vi "Upload VASP File2.vi"(8 "Upload DOS?":bool, 10 "connection reference":T1, 11 "Directory to upload":path=path "C:/Users/Chris B/Documents/Ab Initio/Vasp Calculations/Batch4_20130519/1_Again") -> (3 "IDs":T2)   [LabVIEW 2010]
uses:
  <vilib>/addons/database/NI_Database_API.lvlib
  <vilib>/Analysis/NI_AALBase.lvlib
  <vilib>/Analysis/NI_AALPro.lvlib
  <vilib>/Analysis/_algsub.llb/Real Vector Norm.vi
  <vilib>/Utility/error.llb/DialogType.ctl
  <vilib>/addons/database/Connection.llb/DB Tools Open Connec (Path).vi
  <vilib>/addons/database/Connection.llb/Conn Get Properties.vi
  <vilib>/Utility/file.llb/Read From Spreadsheet File (string).vi
  <vilib>/Analysis/baseanly.llb/Real Dot Product.vi
  <vilib>/addons/database/Connection.llb/Conn ObjectReference.ctl
panel:
  out "INCAR ID":string
  in  "Show Errors?":bool
  out "README":bool
  out "# of atoms":i32
  out "CONTCAR":T3
  out "POSCAR":T3
  out "OUTCAR":bool
  out "DOSCAR":bool
  out "CONTCAR":bool
  out "POSCAR":bool
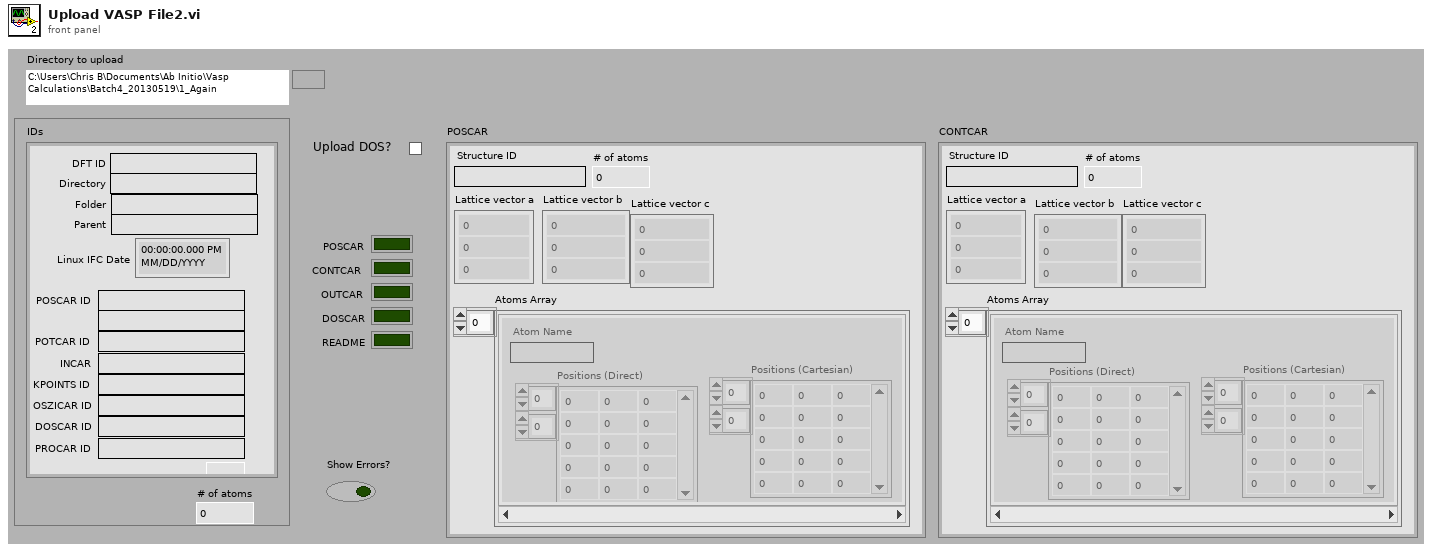
[diagram p1: front panel]
types:
  T1 = typedef "NI_Database_API.lvlib/Conn ObjectReference.ctl" = refnum<k1>
  T2 = cluster{"DFT ID":string, "Directory":string, "Folder":string, "Parent":string, "Linux IFC Date":timestamp, "POSCAR ID":string, "CONTCAR ID":string, "POTCAR ID":string, "INCAR":string, "KPOINTS ID":string, "OSZICAR ID":string, "DOSCAR ID":string, "PROCAR ID":string, "Calc time (Hrs)":dbl}
  T3 = cluster{"Structure ID":string, "Lattice vector a":dbl[], "Lattice vector b":dbl[], "Lattice vector c":dbl[], "Atoms Array":cluster{"Atom Name":string, "Positions (Direct)":dbl[][], "Positions (Cartesian)":dbl[][]}[], "# of atoms":i32}
  T4 = cluster{"Command":string, "Value":string, "Comment":string}[]
  T5 = cluster{"INCAR ID":string, "IBRION":string, "ISIF":string, "ISMEAR":string, "ISPIN":string, "Net Charge":i32}
  T6 = cluster{"INCAR ID":string, "Command":string, "Value":string, "Comment":string}
  T7 = typedef "DialogType.ctl" = u16
  T8 = cluster{"Structure Name":string, "Lattice vector a":dbl[], "Lattice vector b":dbl[], "Lattice vector c":dbl[], "Atoms Array":cluster{"Atom Name":string, "Positions (Direct)":dbl[][], "Positions (Cartesian)":dbl[][]}[], "# of atoms":i32}
  T9 = cluster{"MD5 message-digest":string, string, "name":string, "name":string, "Relaxation Time":timestamp, "Structure ID":string, "Structure ID":string, "MD5 message-digest":string, "INCAR ID":string, "MD5 message-digest":string, "MD5 message-digest":string, "MD5 message-digest":string, "MD5 message-digest":string, "Calc Time (Hrs)":dbl}
  T10 = cluster{"Atom Name":string, "Positions (Direct)":dbl[][], "Positions (Cartesian)":dbl[][]}[]
  T11 = cluster{"[0]":string, "[1]":string, "[2]":string, "[3]":string, "[4]":string, "[5]":string, "[6]":string, "[7]":string, "[8]":string, "[9]":string, "[10]":string, "[11]":string, "[12]":string, "[13]":string, "[14]":string, "[15]":string, "[16]":string, "[17]":string}
  T12 = cluster{"Structure ID":string, "Atom Name":string, "Numeric":dbl, "Numeric":dbl, "Numeric":dbl}
  T13 = cluster{"POTCAR ID":string, "trimmed string":string}
  T14 = cluster{"OSZICAR data":cluster{"Total Free Energy (eV)":dbl, "E0 at Sigma=0 (eV)":dbl, "dE (eV)":dbl, "Electronic Relaxation":dbl[][]}[], "Ionic Relaxation Energies Array (eV)":dbl[], "Bulk Formation Energies Array (eV)":dbl[]}
  T15 = cluster{"Final Energy (eV)":dbl, "Final Energy/atom (eV/atom)":dbl, "Total Formation Energy (eV)":dbl}
  T16 = cluster{"OSZICAR ID":string, "Final Energy (eV)":dbl, "Final Energy/atom (eV/atom)":dbl, "Total Formation Energy (eV)":dbl, i32}
  T17 = cluster{"Energy (eV)":dbl[], "Total DOS":dbl[], "Integrated DOS":dbl[]}
  T18 = cluster{"Fermi Level (eV)":dbl, "# States":dbl, "Density of Valence Band":dbl, "Density of Condution Band":dbl}
  T19 = cluster{"DOSCAR ID":string, "Energy (eV)":dbl[], "Total DOS":dbl[], "Integrated DOS":dbl[], void}
  T20 = cluster{"DOSCAR ID":string, i32, void, void, void}
  T21 = cluster{"DFT ID":string, "String":string, "String":string}
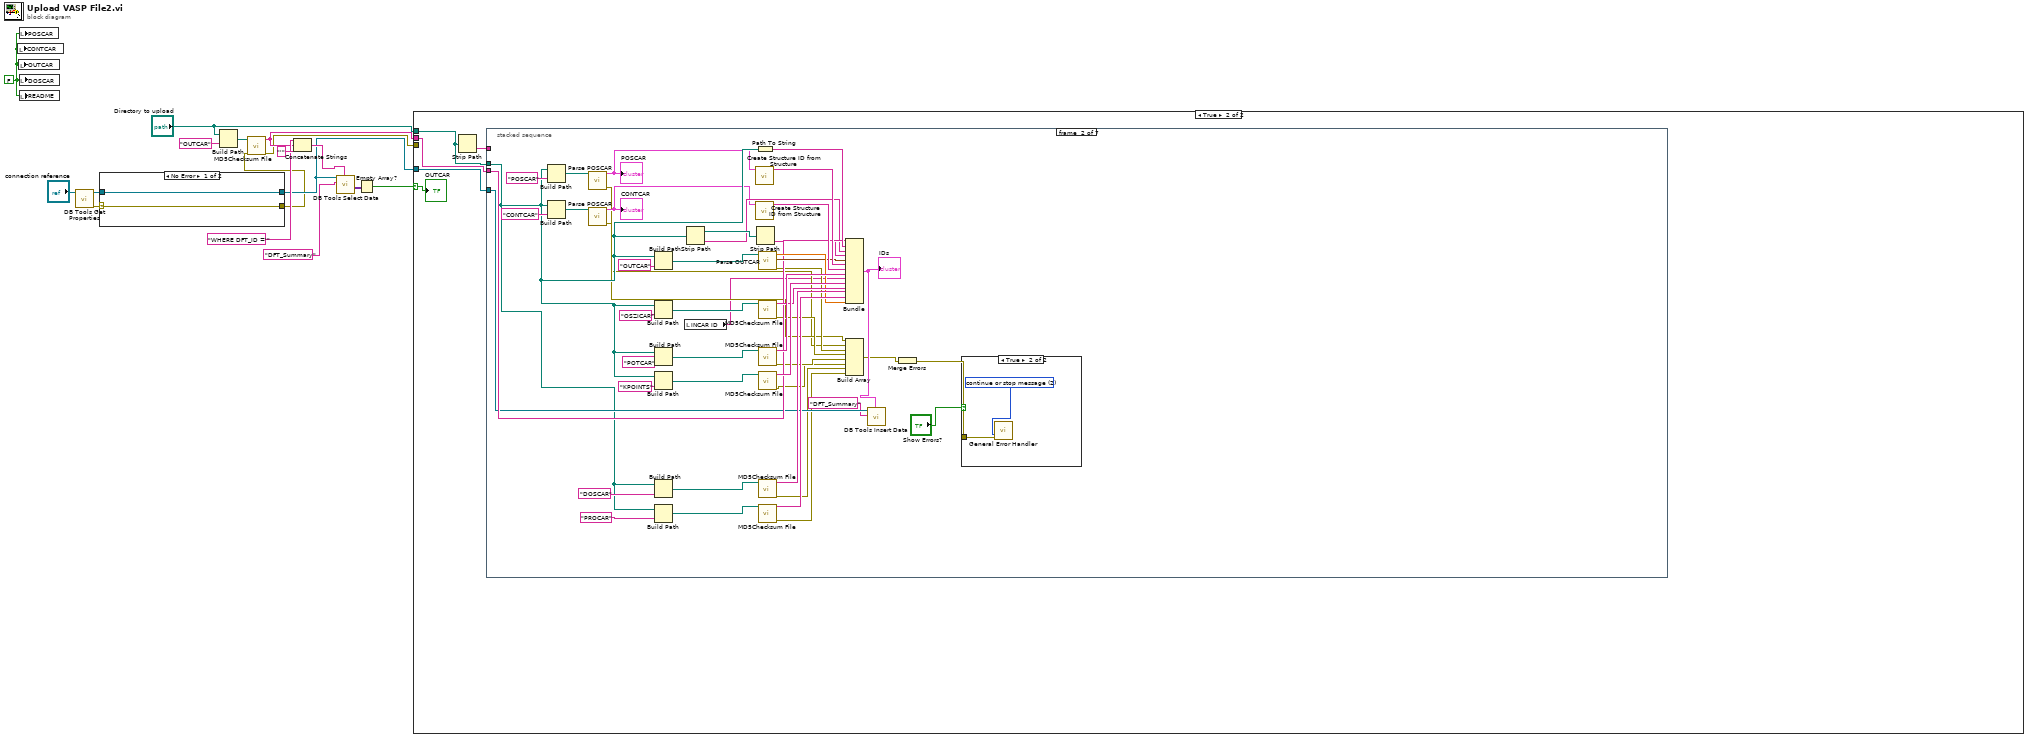
[diagram p0: block diagram]
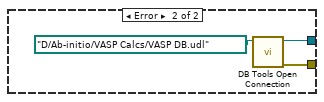
[diagram p2: hidden frame]
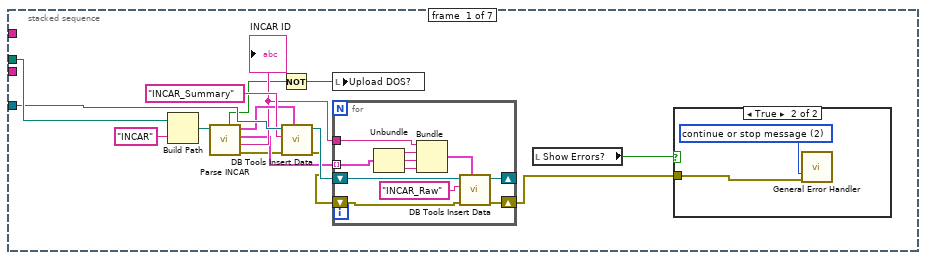
[diagram p4: hidden frame]
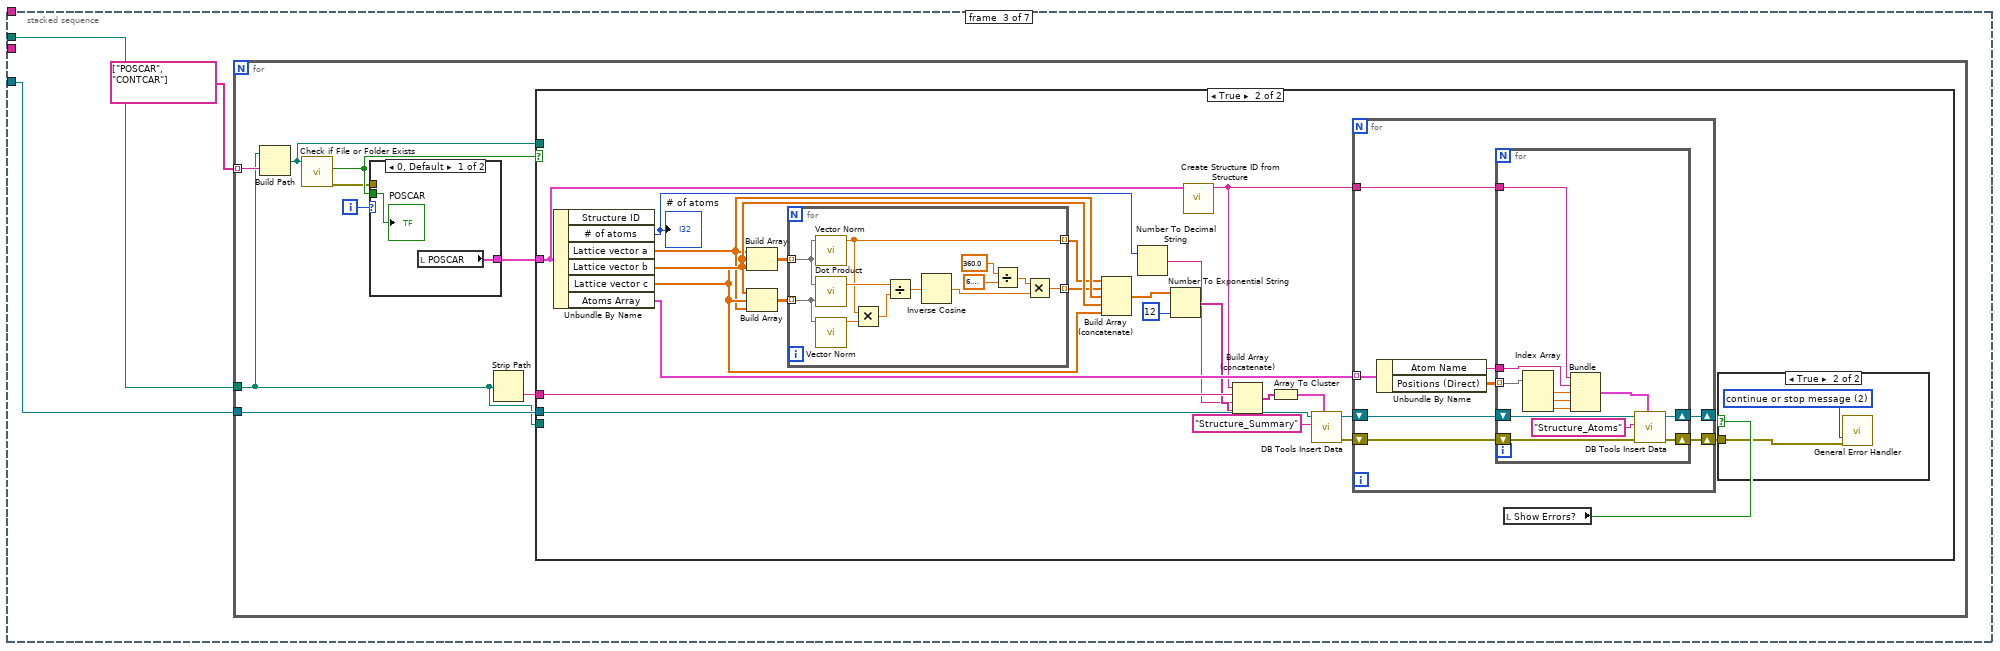
[diagram p7: hidden frame]
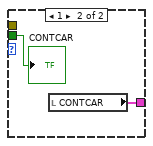
[diagram p10: hidden frame]
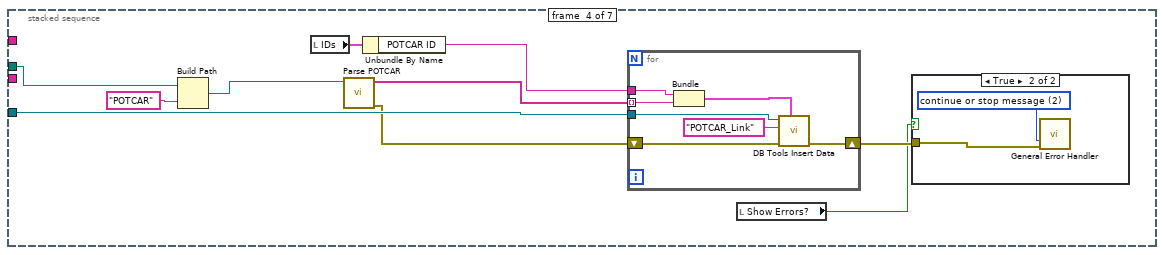
[diagram p11: hidden frame]
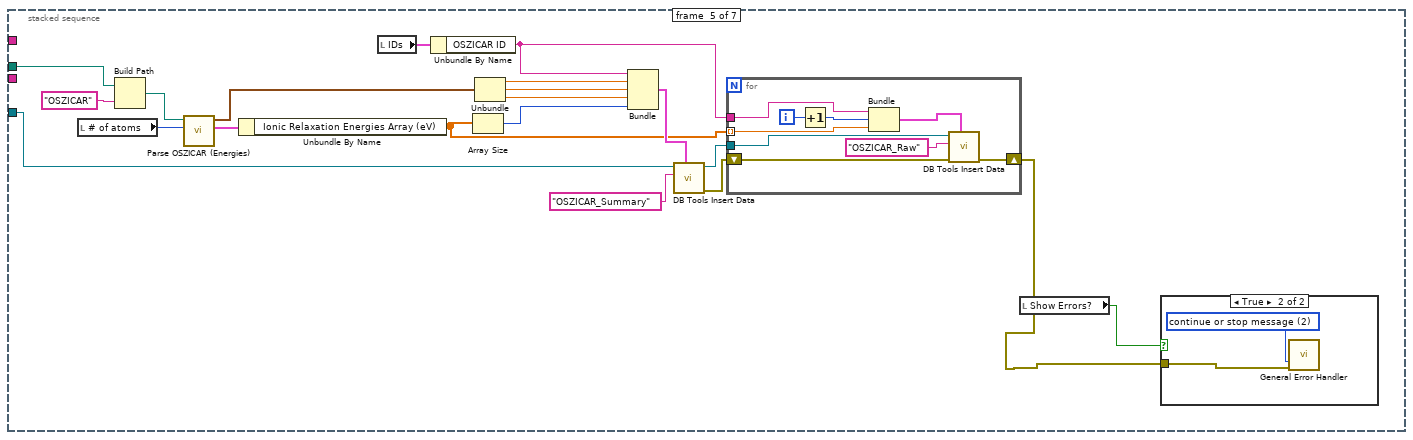
[diagram p13: hidden frame]
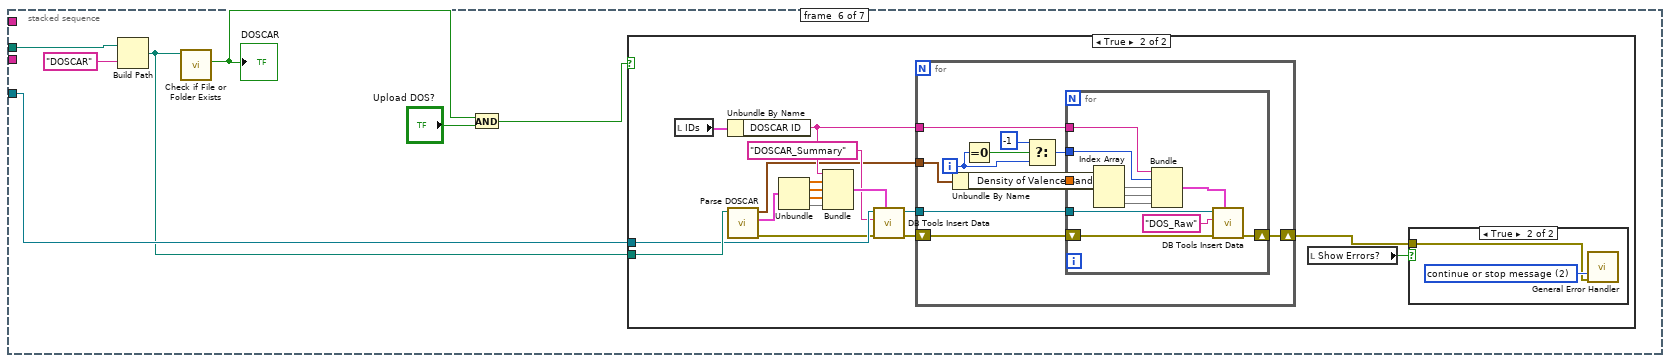
[diagram p15: hidden frame]
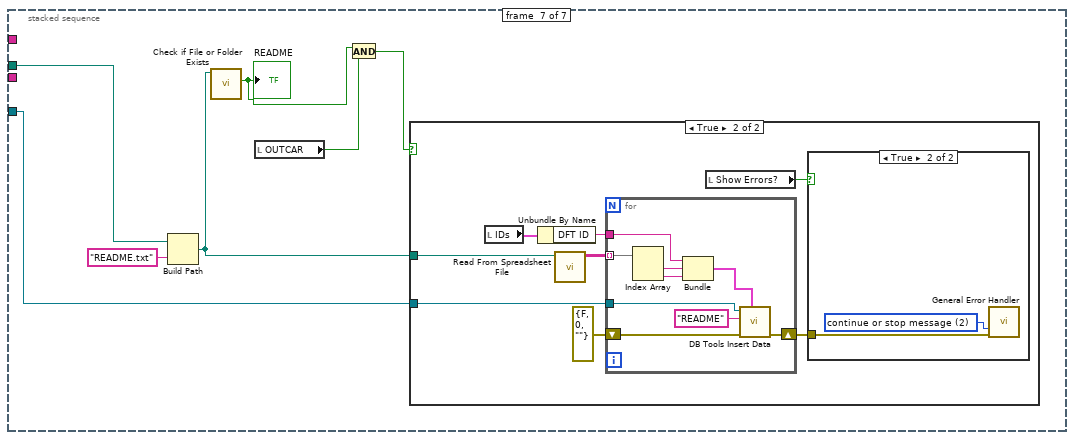
[diagram p18: hidden frame]
diagram:
  w8 = FALSE
  n1 = local write "CONTCAR"(w8) -> ()
  n2 = local write "OUTCAR"(w8) -> ()
  n3 = local write "POSCAR"(w8) -> ()
  n4 = local write "DOSCAR"(w8) -> ()
  n5 = local write "README"(w8) -> ()
  n6 = call-poly <vilib>:"DB Tools Get Properties.vi"("connection reference"="connection reference") -> ("error out"=w5:errorcluster, "connection reference out"=w4:T1)  [unwired: 4 in, 1 out]
  n7 = case shown="No Error" w5 {
    selector: w5 -> [w18 _]
    tunnel: w4 -> [w19 _]
    tunnel: [w19 w22] -> w3
    tunnel: [w18 w20] -> w2
    frame No Error {
    }
    frame Error {
      n8 = call-poly <vilib>:"DB Tools Open Connection.vi"("connection information"=path "D:/Ab-initio/VASP Calcs/VASP DB.udl" ("UDL")) -> ("error out"=w20:errorcluster, "connection reference"=w22:T1)  [unwired: 7 in]
    }
  }
  n9 = Build Path(base path="Directory to upload", name or relative path="OUTCAR") -> (appended path=w13:path)
  n10 = call <vilib>:"MD5Checksum File.vi"("error in (no error)"=w2, "Path"=w13) -> ("error out"=w7:errorcluster, "MD5 message-digest"=w11:string)  [unwired: 8 in]
  n11 = Concatenate Strings("WHERE DFT_ID ='" ("string"), w11, "'" ("string")) -> (w17:string)
  n12 = call <vilib>:"DB Tools Select Data.vi"("condition"=w17, "table"="DFT_Summary", "connection reference"=w3) -> ("data"=w1:variant[][])  [unwired: 3 in, 2 out]
  n13 = Empty Array?(array=w1) -> (empty?=w9:bool)
  n14 = case shown="True" w9 {
    selector: w9 -> [_ w23]
    tunnel: w11 -> [_ w26]
    tunnel: w3 -> [_ w25]
    tunnel: "Directory to upload" -> [_ w24]
    tunnel: w7 -> [_ _]
    frame False {
    }
    frame True {
      n15 = Strip Path(path=w24) -> (name=w27:string)  [unwired: 1 out]
      n16 = stacked-sequence {
        tunnel: w24 -> [w42 w75 w108 w189 w217 w236 w282]
        tunnel: w25 -> [w38 w76 w107 w183 w206 w235 w281]
        tunnel: w27 -> [_ _ _ _ _ _ _]
        tunnel: w26 -> [_ w77 _ _ _ _ _]
        frame #0 {
          n17 = Build Path(base path=w42, name or relative path="INCAR") -> (appended path=w40:path)
          n18 = call "Parse INCAR.vi"("INCAR File"=w40) -> ("error out"=w31:errorcluster, "INCAR ID"=w34:string, "INCAR Raw Commands"=w33:T4, "INCAR Summary"=w35:T5, "Allow Relaxation?"=w32:bool)  [unwired: 6 in]
          "INCAR ID" <- w34
          n19 = Not(x=w32) -> (.not. x?=w39:bool)
          n20 = call <vilib>:"DB Tools Insert Data.vi"("data"=w35, "error in (no error)"=w31, "table"="INCAR_Summary", "connection reference"=w38) -> ("error out"=w29:errorcluster, "connection reference out"=w37:T1)  [unwired: 6 in]
          n21 = local write "Upload DOS?"(w39) -> ()
          n22 = for {
            tunnel: w33 -> [w55] mode=indexing
            tunnel: w34 -> [w48]
            shift-right: [w53] -> _
            shift-left: w37 -> [w54]
            shift-right: [w46] -> w28
            shift-left: w29 -> [w45]
            n23 = Unbundle(w55) -> ("Command"=w52:string, "Value"=w51:string, "Comment"=w50:string)
            n24 = Bundle("INCAR ID"=w48, "Command"=w52, "Value"=w51, "Comment"=w50) -> (w49:T6)  [unwired: 1 in]
            n25 = call <vilib>:"DB Tools Insert Data.vi"("data"=w49, "error in (no error)"=w45, "table"="INCAR_Raw", "connection reference"=w54) -> ("error out"=w46:errorcluster, "connection reference out"=w53:T1)  [unwired: 6 in]
          }
          n26 = local read "Show Errors?"() -> (w30:bool)
          n27 = case shown="True" w30 {
            tunnel: w28 -> [_ w44]
            frame False {
            }
            frame True {
              w43 = T7 2 items=["no dialog", "OK message", "continue or stop message", "OK message + warnings", "continue/stop + warnings"] ("type of dialog (OK msg:1)")
              n28 = call <vilib>:"General Error Handler.vi"("type of dialog (OK msg:1)"=w43, "error in (no error)"=w44) -> ()  [unwired: 9 in, 5 out]
            }
          }
        }
        frame #1 {
          n29 = Build Path(base path=w75, name or relative path="POSCAR") -> (appended path=w97:path)
          n30 = Build Path(base path=w75, name or relative path="CONTCAR") -> (appended path=w96:path)
          n31 = call "Parse POSCAR.vi"("POSCAR File"=w97) -> ("error out"=w61:errorcluster, "Structure"=w63:T8)  [unwired: 7 in, 2 out]
          "POSCAR" <- w63
          n32 = call "Parse POSCAR.vi"("POSCAR File"=w96) -> ("error out"=w60:errorcluster, "Structure"=w62:T8)  [unwired: 7 in, 2 out]
          "CONTCAR" <- w62
          n33 = Build Path(base path=w75, name or relative path="OUTCAR") -> (appended path=w102:path)
          n34 = Build Path(base path=w75, name or relative path="OSZICAR") -> (appended path=w89:path)
          n35 = Build Path(base path=w75, name or relative path="POTCAR") -> (appended path=w100:path)
          n36 = Build Path(base path=w75, name or relative path="KPOINTS") -> (appended path=w90:path)
          n37 = Build Path(base path=w75, name or relative path="DOSCAR") -> (appended path=w83:path)
          n38 = Build Path(base path=w75, name or relative path="PROCAR") -> (appended path=w84:path)
          n39 = local read "INCAR ID"() -> (w56:string)
          n40 = Strip Path(path=w75) -> (stripped path=w74:path, name=w73:string)
          n41 = call "Create Structure ID from Structure.vi"("Structure"=w63) -> ("Structure ID"=w94:string)  [unwired: 10 in]
          n42 = call "Create Structure ID from Structure.vi"("Structure"=w62) -> ("Structure ID"=w93:string)  [unwired: 10 in]
          n43 = Path To String(path=w75) -> (string=w95:string)
          n44 = Strip Path(path=w74) -> (name=w72:string)  [unwired: 1 out]
          n45 = call "Parse OUTCAR.vi"("OUTCAR File"=w102) -> ("error out"=w64:errorcluster, "Relaxation Time"=w78:timestamp, "Calc Time (Hrs)"=w79:dbl)  [unwired: 8 in]
          n46 = call <vilib>:"MD5Checksum File.vi"("Path"=w89) -> ("error out"=w69:errorcluster, "MD5 message-digest"=w86:string)  [unwired: 9 in]
          n47 = call <vilib>:"MD5Checksum File.vi"("Path"=w100) -> ("error out"=w68:errorcluster, "MD5 message-digest"=w92:string)  [unwired: 9 in]
          n48 = call <vilib>:"MD5Checksum File.vi"("Path"=w90) -> ("error out"=w67:errorcluster, "MD5 message-digest"=w87:string)  [unwired: 9 in]
          n49 = call <vilib>:"MD5Checksum File.vi"("Path"=w83) -> ("error out"=w66:errorcluster, "MD5 message-digest"=w81:string)  [unwired: 9 in]
          n50 = call <vilib>:"MD5Checksum File.vi"("Path"=w84) -> ("error out"=w65:errorcluster, "MD5 message-digest"=w80:string)  [unwired: 9 in]
          n51 = Bundle("MD5 message-digest"=w77, w95, "name"=w73, "name"=w72, "Relaxation Time"=w78, "Structure ID"=w94, "Structure ID"=w93, "MD5 message-digest"=w92, "INCAR ID"=w56, "MD5 message-digest"=w87, "MD5 message-digest"=w86, "MD5 message-digest"=w81, "MD5 message-digest"=w80, "Calc Time (Hrs)"=w79) -> (w70:T9)  [unwired: 1 in]
          "IDs" <- w70
          n52 = Build Array(w61, w60, w64, w69, w68, w67, w66, w65) -> (w59:errorcluster[])
          n53 = call <vilib>:"DB Tools Insert Data.vi"("data"=w70, "table"="DFT_Summary", "connection reference"=w76) -> ()  [unwired: 7 in, 2 out]
          n54 = Merge Errors(w59) -> (w57:errorcluster)
          n55 = case shown="True" "Show Errors?" {
            tunnel: w57 -> [_ w105]
            frame False {
            }
            frame True {
              w104 = T7 2 items=["no dialog", "OK message", "continue or stop message", "OK message + warnings", "continue/stop + warnings"] ("type of dialog (OK msg:1)")
              n56 = call <vilib>:"General Error Handler.vi"("type of dialog (OK msg:1)"=w104, "error in (no error)"=w105) -> ()  [unwired: 9 in, 5 out]
            }
          }
        }
        frame #2 {
          n57 = for {
            tunnel: string[] ["POSCAR", "CONTCAR"] -> [w116] mode=indexing
            tunnel: w108 -> [w112]
            tunnel: w107 -> [w117]
            i -> [w114]
            n58 = Build Path(base path=w112, name or relative path=w116) -> (appended path=w115:path)
            n59 = call <vilib>:"Check if File or Folder Exists.vi"("path"=w115) -> ("error out"=w109:errorcluster, "file or folder exists?"=w113:bool)  [unwired: 8 in, 1 out]
            n60 = case shown="0, Default" w114 {
              tunnel: w113 -> [w177 w179]
              tunnel: [w176 w178] -> w110
              tunnel: w109 -> [_ _]
              frame 0, Default {
                n61 = local read "POSCAR"() -> (w176:T3)
                "POSCAR" <- w177
              }
              frame 1 {
                n62 = local read "CONTCAR"() -> (w178:T3)
                "CONTCAR" <- w179
              }
            }
            n63 = Strip Path(path=w112) -> (name=w111:string)  [unwired: 1 out]
            n64 = case shown="True" w113 {
              tunnel: w117 -> [_ w141]
              tunnel: w112 -> [_ _]
              tunnel: w115 -> [_ _]
              tunnel: w111 -> [_ w140]
              tunnel: w110 -> [_ w123]
              frame False {
              }
              frame True {
                n65 = Unbundle By Name(w123) -> ("# of atoms"=w118:i32, "Lattice vector a"=w136:dbl[], "Lattice vector b"=w138:dbl[], "Lattice vector c"=w137:dbl[], "Atoms Array"=w127:T10)  [unwired: 1 out]
                "# of atoms" <- w118
                n66 = Build Array(w136, w138, w137) -> (w139:dbl[][])
                n67 = Build Array(w138, w137, w136) -> (w135:dbl[][])
                n68 = for {
                  tunnel: w139 -> [w174] mode=indexing
                  tunnel: w135 -> [w173] mode=indexing
                  tunnel: [w169] -> w134 mode=indexing
                  tunnel: [w165] -> w133 mode=indexing
                  n69 = call-poly <vilib>:"Vector Norm.vi"("Input Vector"=w174) -> ("norm"=w169:dbl)  [unwired: 9 in, 1 out]
                  n70 = call-poly <vilib>:"Dot Product.vi"("Y Vector"=w173, "X Vector"=w174) -> ("X * Y"=w175:dbl)  [unwired: 1 out]
                  n71 = call-poly <vilib>:"Vector Norm.vi"("Input Vector"=w173) -> ("norm"=w172:dbl)  [unwired: 9 in, 1 out]
                  n72 = Multiply(x=w169, y=w172) -> (x*y=w171:dbl)
                  n73 = Divide(x=w175, y=w171) -> (x/y=w170:dbl)
                  n74 = Inverse Cosine(1:w170) -> (0:w166:dbl)
                  n75 = Divide(x=360.0, y=6.283185307179586) -> (x/y=w167:dbl)
                  n76 = Multiply(x=w167, y=w166) -> (x*y=w165:dbl)
                }
                n77 = Build Array (concatenate)(w134, w133, w136, w138, w137) -> (w132:dbl[])
                n78 = Number To Decimal String(number=w118) -> (decimal integer string=w119:string)  [unwired: 1 in]
                n79 = Number To Exponential String(number=w132, precision (6)=i16 12) -> (E-format string=w120:string[])  [unwired: 2 in]
                n80 = call "Create Structure ID from Structure.vi"("Structure"=w123) -> ("Structure ID"=w124:string)  [unwired: 10 in]
                n81 = Build Array (concatenate)(w124, w140, w119, w120) -> (w130:string[])
                n82 = Array To Cluster(array=w130) -> (cluster=w129:T11)
                n83 = call <vilib>:"DB Tools Insert Data.vi"("data"=w129, "table"="Structure_Summary", "connection reference"=w141) -> ("error out"=w126:errorcluster, "connection reference out"=w125:T1)  [unwired: 7 in]
                n84 = for {
                  tunnel: w127 -> [w151] mode=indexing
                  shift-right: [w148] -> w121
                  shift-left: w126 -> [w149]
                  shift-right: [w147] -> _
                  shift-left: w125 -> [w150]
                  tunnel: w124 -> [w144]
                  n85 = Unbundle By Name(w151) -> ("Atom Name"=w146:string, "Positions (Direct)"=w145:dbl[][])
                  n86 = for {
                    shift-right: [w162] -> w147
                    shift-left: w150 -> [w163]
                    shift-right: [w160] -> w148
                    shift-left: w149 -> [w161]
                    tunnel: w146 -> [w159]
                    tunnel: w145 -> [w157] mode=indexing
                    tunnel: w144 -> [w158]
                    n87 = Index Array(array=w157) -> (element #1=w156:dbl, element #2=w155:dbl, element #3=w154:dbl)  [unwired: 3 in]
                    n88 = Bundle("Structure ID"=w158, "Atom Name"=w159, "Numeric"=w156, "Numeric"=w155, "Numeric"=w154) -> (w153:T12)  [unwired: 1 in]
                    n89 = call <vilib>:"DB Tools Insert Data.vi"("data"=w153, "error in (no error)"=w161, "table"="Structure_Atoms", "connection reference"=w163) -> ("error out"=w160:errorcluster, "connection reference out"=w162:T1)  [unwired: 6 in]
                  }
                }
                n90 = local read "Show Errors?"() -> (w122:bool)
                n91 = case shown="True" w122 {
                  tunnel: w121 -> [_ w143]
                  frame False {
                  }
                  frame True {
                    w142 = T7 2 items=["no dialog", "OK message", "continue or stop message", "OK message + warnings", "continue/stop + warnings"] ("type of dialog (OK msg:1)")
                    n92 = call <vilib>:"General Error Handler.vi"("type of dialog (OK msg:1)"=w142, "error in (no error)"=w143) -> ()  [unwired: 9 in, 5 out]
                  }
                }
              }
            }
          }
        }
        frame #3 {
          n93 = Build Path(base path=w189, name or relative path="POTCAR") -> (appended path=w187:path)
          n94 = local read "IDs"() -> (w186:T2)
          n95 = call "Parse POTCAR.vi"("POTCAR File"=w187) -> ("error out"=w182:errorcluster, "POTCARs"=w185:string[])  [unwired: 9 in]
          n96 = Unbundle By Name(w186) -> ("POTCAR ID"=w184:string)
          n97 = for {
            tunnel: w185 -> [w198] mode=indexing
            tunnel: w184 -> [w197]
            tunnel: w183 -> [w194]
            shift-right: [w193] -> w181
            shift-left: w182 -> [w192]
            n98 = Bundle("POTCAR ID"=w197, "trimmed string"=w198) -> (w196:T13)  [unwired: 1 in]
            n99 = call <vilib>:"DB Tools Insert Data.vi"("data"=w196, "error in (no error)"=w192, "table"="POTCAR_Link", "connection reference"=w194) -> ("error out"=w193:errorcluster)  [unwired: 6 in, 1 out]
          }
          n100 = local read "Show Errors?"() -> (w180:bool)
          n101 = case shown="True" w180 {
            tunnel: w181 -> [_ w191]
            frame False {
            }
            frame True {
              w190 = T7 2 items=["no dialog", "OK message", "continue or stop message", "OK message + warnings", "continue/stop + warnings"] ("type of dialog (OK msg:1)")
              n102 = call <vilib>:"General Error Handler.vi"("type of dialog (OK msg:1)"=w190, "error in (no error)"=w191) -> ()  [unwired: 9 in, 5 out]
            }
          }
        }
        frame #4 {
          n103 = local read "# of atoms"() -> (w215:i32)
          n104 = Build Path(base path=w217, name or relative path="OSZICAR") -> (appended path=w216:path)
          n105 = call "Parse OSZICAR (Energies).vi"("# of Atoms"=w215, "OSZICAR File"=w216) -> ("OSZICAR Raw"=w213:T14, "Extracted Parameters"=w212:T15)  [unwired: 6 in, 2 out]
          n106 = Unbundle By Name(w213) -> ("Ionic Relaxation Energies Array (eV)"=w203:dbl[])
          n107 = local read "IDs"() -> (w214:T2)
          n108 = Unbundle By Name(w214) -> ("OSZICAR ID"=w202:string)
          n109 = Array Size(array=w203) -> (size(s)=w208:i32)
          n110 = Unbundle(w212) -> ("Final Energy (eV)"=w211:dbl, "Final Energy/atom (eV/atom)"=w210:dbl, "Total Formation Energy (eV)"=w209:dbl)
          n111 = Bundle("OSZICAR ID"=w202, "Final Energy (eV)"=w211, "Final Energy/atom (eV/atom)"=w210, "Total Formation Energy (eV)"=w209, w208) -> (w207:T16)  [unwired: 1 in]
          n112 = call <vilib>:"DB Tools Insert Data.vi"("data"=w207, "table"="OSZICAR_Summary", "connection reference"=w206) -> ("error out"=w204:errorcluster, "connection reference out"=w205:T1)  [unwired: 7 in]
          n113 = for {
            tunnel: w205 -> [w229]
            shift-right: [w227] -> w199
            shift-left: w204 -> [w226]
            tunnel: w203 -> [w222] mode=indexing
            tunnel: w202 -> [w223]
            i -> [w225]
            n114 = Increment(x=w225) -> (x+1=w224:i32)
            n115 = Bundle("OSZICAR ID"=w223, w224, w222) -> (w221:cluster{"OSZICAR ID":string, i32, dbl})  [unwired: 1 in]
            n116 = call <vilib>:"DB Tools Insert Data.vi"("data"=w221, "error in (no error)"=w226, "table"="OSZICAR_Raw", "connection reference"=w229) -> ("error out"=w227:errorcluster)  [unwired: 6 in, 1 out]
          }
          n117 = local read "Show Errors?"() -> (w200:bool)
          n118 = case shown="True" w200 {
            tunnel: w199 -> [_ w220]
            frame False {
            }
            frame True {
              w219 = T7 2 items=["no dialog", "OK message", "continue or stop message", "OK message + warnings", "continue/stop + warnings"] ("type of dialog (OK msg:1)")
              n119 = call <vilib>:"General Error Handler.vi"("type of dialog (OK msg:1)"=w219, "error in (no error)"=w220) -> ()  [unwired: 9 in, 5 out]
            }
          }
        }
        frame #5 {
          n120 = Build Path(base path=w236, name or relative path="DOSCAR") -> (appended path=w233:path)
          n121 = call <vilib>:"Check if File or Folder Exists.vi"("path"=w233) -> ("file or folder exists?"=w231:bool)  [unwired: 8 in, 2 out]
          "DOSCAR" <- w231
          n122 = And(x=w231, y="Upload DOS?") -> (x .and. y?=w232:bool)
          n123 = case shown="True" w232 {
            tunnel: w235 -> [_ w244]
            tunnel: w233 -> [_ w253]
            frame False {
            }
            frame True {
              n124 = local read "IDs"() -> (w252:T2)
              n125 = Unbundle By Name(w252) -> ("DOSCAR ID"=w250:string)
              n126 = call "Parse DOSCAR.vi"("Path"=w253) -> ("error out"=w239:errorcluster, "Total DOS"=w251:T17, "DOS Summary"=w240:T18)  [unwired: 7 in, 1 out]
              n127 = Unbundle(w251) -> (w249:dbl[], w248:dbl[], w246:dbl[], w247)
              n128 = Bundle("DOSCAR ID"=w250, "Energy (eV)"=w249, "Total DOS"=w248, "Integrated DOS"=w246, w247) -> (w245:T19)  [unwired: 1 in]
              n129 = call <vilib>:"DB Tools Insert Data.vi"("data"=w245, "error in (no error)"=w239, "table"="DOSCAR_Summary", "connection reference"=w244) -> ("error out"=w242:errorcluster, "connection reference out"=w243:T1)  [unwired: 6 in]
              n130 = for {
                tunnel: w243 -> [w263]
                tunnel: w250 -> [w264]
                shift-right: [w262] -> w238
                shift-left: w242 -> [w261]
                tunnel: w240 -> [w260]
                i -> [w257]
                n131 = Unbundle By Name(w260) -> ("Density of Valence Band"=w259:dbl)
                n132 = Equal To 0?(x=w257) -> (x = 0?=w265:bool)
                n133 = Select(t=-1, s=w265, f=w257) -> (s? t:f=w256:i32)
                n134 = for {
                  tunnel: w264 -> [w274]
                  tunnel: w256 -> [w273]
                  tunnel: w259 -> [w272]
                  tunnel: w263 -> [w275]
                  shift-right: [w267] -> w262
                  shift-left: w261 -> [w266]
                  n135 = Index Array(array=w272) -> (element #1=w271, element #2=w270, element #3=w269)  [unwired: 3 in]
                  n136 = Bundle("DOSCAR ID"=w274, w273, w271, w270, w269) -> (w268:T20)  [unwired: 1 in]
                  n137 = call <vilib>:"DB Tools Insert Data.vi"("data"=w268, "error in (no error)"=w266, "table"="DOS_Raw", "connection reference"=w275) -> ("error out"=w267:errorcluster)  [unwired: 6 in, 1 out]
                }
              }
              n138 = local read "Show Errors?"() -> (w237:bool)
              n139 = case shown="True" w237 {
                tunnel: w238 -> [_ w254]
                frame False {
                }
                frame True {
                  w255 = T7 2 items=["no dialog", "OK message", "continue or stop message", "OK message + warnings", "continue/stop + warnings"] ("type of dialog (OK msg:1)")
                  n140 = call <vilib>:"General Error Handler.vi"("type of dialog (OK msg:1)"=w255, "error in (no error)"=w254) -> ()  [unwired: 9 in, 5 out]
                }
              }
            }
          }
        }
        frame #6 {
          n141 = Build Path(base path=w282, name or relative path="README.txt") -> (appended path=w280:path)
          n142 = call <vilib>:"Check if File or Folder Exists.vi"("path"=w280) -> ("file or folder exists?"=w279:bool)  [unwired: 8 in, 2 out]
          "README" <- w279
          n143 = local read "OUTCAR"() -> (w277:bool)
          n144 = And(x=w279, y=w277) -> (x .and. y?=w278:bool)
          n145 = case shown="True" w278 {
            tunnel: w281 -> [_ w288]
            tunnel: w280 -> [_ w286]
            frame False {
            }
            frame True {
              n146 = local read "IDs"() -> (w291:T2)
              n147 = Unbundle By Name(w291) -> ("DFT ID"=w289:string)
              n148 = call-poly <vilib>:"Read From Spreadsheet File.vi"("file path (dialog if empty)"=w286) -> ("all rows"=w290:string[][])  [unwired: 6 in, 4 out]
              n149 = for {
                tunnel: w290 -> [w302] mode=indexing
                tunnel: w289 -> [w301]
                tunnel: w288 -> [w297]
                shift-right: [w296] -> w284
                shift-left: errorcluster {"status"=FALSE, "code"=0, "source"=""} ("error out") -> [w295]
                n150 = Index Array(array=w302) -> (element #1=w300:string, element #2=w299:string)  [unwired: 2 in]
                n151 = Bundle("DFT ID"=w301, "String"=w300, "String"=w299) -> (w298:T21)  [unwired: 1 in]
                n152 = call <vilib>:"DB Tools Insert Data.vi"("data"=w298, "error in (no error)"=w295, "table"="README", "connection reference"=w297) -> ("error out"=w296:errorcluster)  [unwired: 6 in, 1 out]
              }
              n153 = local read "Show Errors?"() -> (w285:bool)
              n154 = case shown="True" w285 {
                tunnel: w284 -> [_ w292]
                frame False {
                }
                frame True {
                  w293 = T7 2 items=["no dialog", "OK message", "continue or stop message", "OK message + warnings", "continue/stop + warnings"] ("type of dialog (OK msg:1)")
                  n155 = call <vilib>:"General Error Handler.vi"("type of dialog (OK msg:1)"=w293, "error in (no error)"=w292) -> ()  [unwired: 9 in, 5 out]
                }
              }
            }
          }
        }
      }
      "OUTCAR" <- w23
    }
  }
